vi "Error Logger.vi"(8 "error in (no error)":errorcluster, 11 "Message":string) -> (0 "error out":errorcluster)   [LabVIEW 2018]
doc: "Logs eeror"
uses:
  <vilib>/Utility/file.llb/Write Delimited Spreadsheet (string).vi
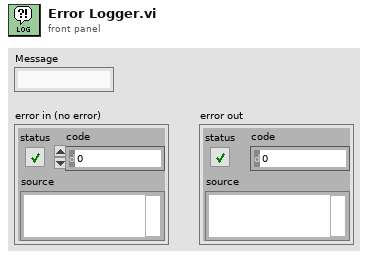
[diagram p1: front panel]
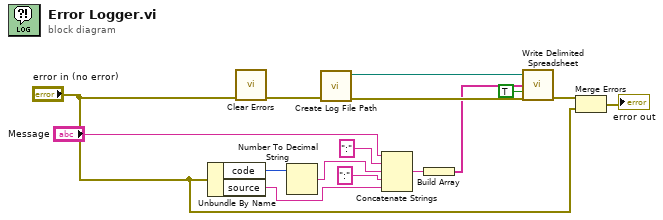
[diagram p0: block diagram]
diagram:
  n1 = Unbundle By Name("error in (no error)") -> ("code"=w5:i32, "source"=w6:string)
  n2 = call <vilib>:"Clear Errors.vi"("error in (no error)"="error in (no error)") -> ("error out"=w11:errorcluster)  [unwired: 5 in, 1 out]
  n3 = Number To Decimal String(number=w5) -> (decimal integer string=w8:string)  [unwired: 1 in]
  n4 = call "Create Log File Path.vi"("error in (no error)"=w11) -> ("error out"=w13:errorcluster, "dup path"=w12:path)  [unwired: 9 in]
  n5 = Concatenate Strings("Message", ":" ("string"), w8, ":" ("string"), w6) -> (w9:string)
  n6 = Build Array(w9) -> (w10:string[])
  n7 = call-poly <vilib>:"Write Delimited Spreadsheet.vi"("file path (dialog if empty)"=w12, "1D data"=w10, "append to file? (new file:F)"=TRUE, "error in (no error)"=w13) -> ("error out"=w3:errorcluster)  [unwired: 10 in, 1 out]
  n8 = Merge Errors(w3, "error in (no error)") -> (→"error out":errorcluster)
